vi "Two Fgen Module T11.vi"() -> ()   [LabVIEW 2021, in "Waveform Generator T11.lvlib"]
uses:
  Waveform Generator T11.lvlib
  controls/Type.ctl
  subVIs/Common Dep T11.lvlib
panel:
  out "Sine Pass?":bool[](array[boolean])
  in  "Sine Wave":refnum<k15>="PXI1Slot2,PXI1Slot3" caption="resource name"
  out "Square Pass?":bool[](array[boolean])
  in  "Square Wave":refnum<k15>="PXI1Slot2,PXI1Slot3" caption="resource name"
  in  "I3C Generator Fgen Channel":string
  in  "I3C waveform":T1(ring)=enum."Noise"
  in  "I3C frequency":dbl=6.0
  in  "I3C amplitude":dbl=6.0
  in  "I3C Generator Fgen":refnum<k15>
  out "I3C Duration":dbl
  in  "duration":dbl
  out "I2C Duration":dbl
  in  "I2C Generator Fgen":refnum<k15>
  in  "I2C amplitude":dbl=6.0
  in  "I2C frequency":dbl=6.0
  in  "I2C waveform":T2=enum."Noise"
  in  "I2C Generator Fgen Channel":string
  out "error out":errorcluster
  in  "error in":errorcluster
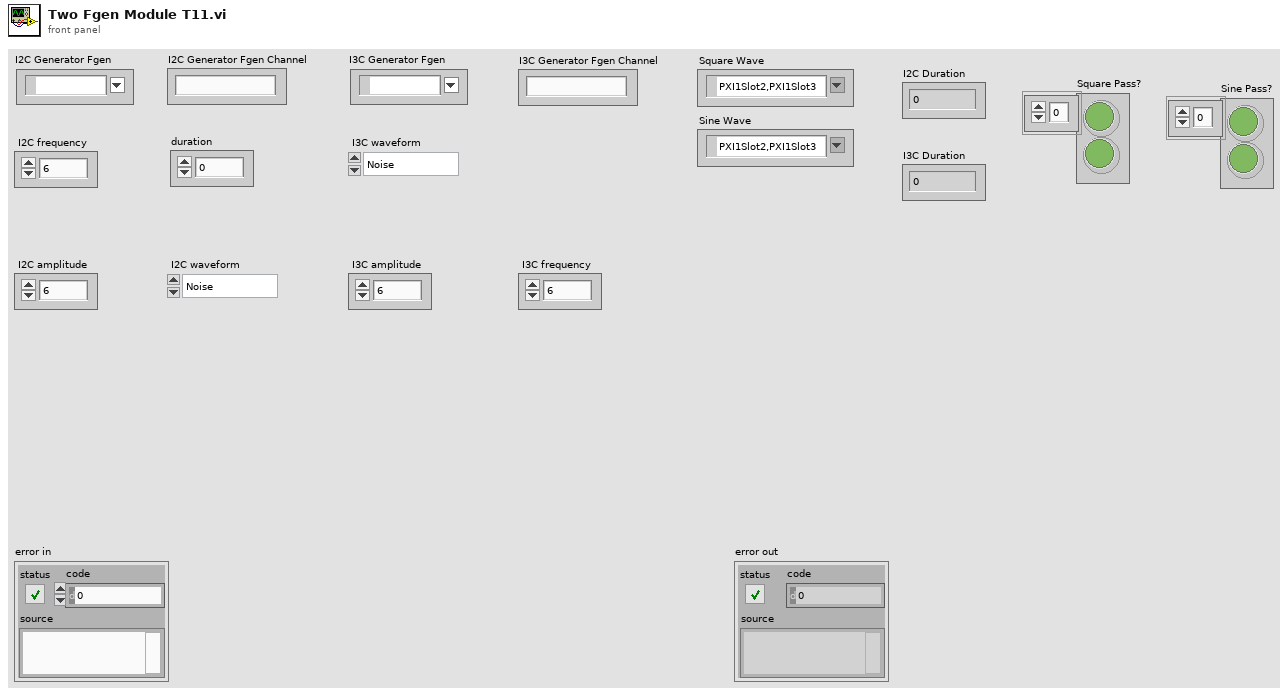
[diagram p1: front panel]
types:
  T1 = enum32{"Sine", "Square", "Triangle", "Ramp Up", "Ramp Down", "DC", "Noise", "User"}
  T2 = typedef "Waveform Generator T11.lvlib/Type.ctl" = enum32{"Sine", "Square", "Triangle", "Ramp Up", "Ramp Down", "DC", "Noise", "User"}
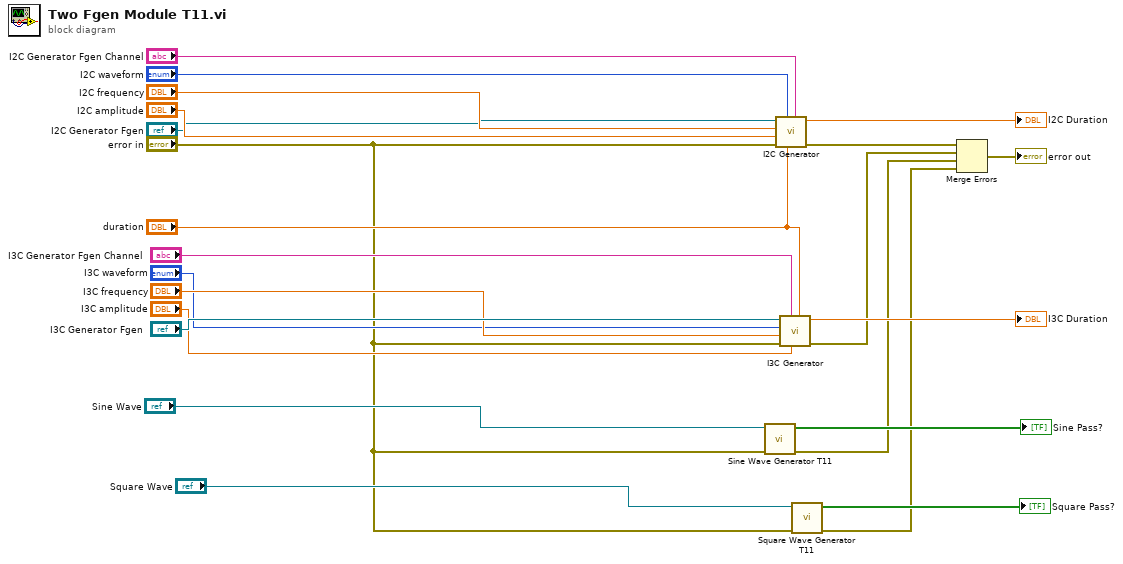
[diagram p0: block diagram]
diagram:
  n1 = call "Sine Wave Generator T11.vi"("error in (no error)"="error in", "IVI Refnum in"="Sine Wave") -> ("error out"=w2:errorcluster, "pass"=→"Sine Pass?":bool[])  [unwired: 8 in]
  n2 = call "I2C Generator.vi"("I2C Generator Fgen Channel"="I2C Generator Fgen Channel", "duration"="duration", "I2C waveform"="I2C waveform", "error in (no error)"="error in", "I2C amplitude"="I2C amplitude", "I2C frequency"="I2C frequency", "IVI Refnum in"="I2C Generator Fgen") -> ("error out"=w23:errorcluster, "Numeric"=→"I2C Duration":dbl)  [unwired: 3 in]
  n3 = call "I3C Generator.vi"("duration"="duration", "I3C amplitude"="I3C amplitude", "I3C Generator Fgen Channel"="I3C Generator Fgen Channel", "error in (no error)"="error in", "I3C frequency"="I3C frequency", "I3C waveform"="I3C waveform", "IVI Refnum in"="I3C Generator Fgen") -> ("error out"=w8:errorcluster, "Numeric"=→"I3C Duration":dbl)  [unwired: 3 in]
  n4 = call "Square Wave Generator T11.vi"("error in (no error)"="error in", "IVI Refnum in"="Square Wave") -> ("error out"=w1:errorcluster, "pass"=→"Square Pass?":bool[])  [unwired: 8 in]
  n5 = Merge Errors(w23, w8, w2, w1) -> (→"error out":errorcluster)
